vi "VI Tree.vi"() -> ()   [LabVIEW 2017]
uses:
  Private/RegisterVI.vi
  Private/RegisterVIs.vi
  API/JKI Simple Localization.lvlib
panel:
  out "Languages":string[](array[string])
  out "Languages":string[](array[string])
  out "Translated Phrase":string
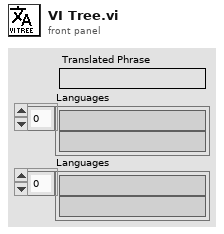
[diagram p1: front panel]
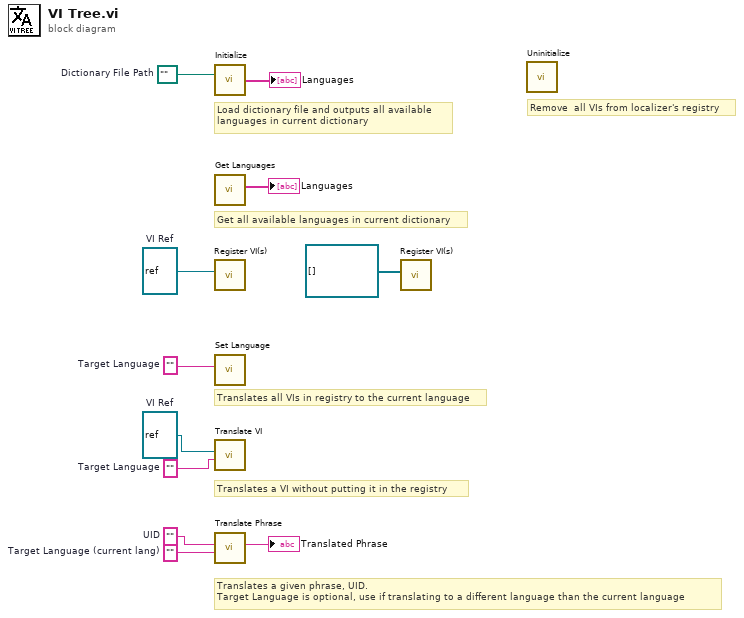
[diagram p0: block diagram]
diagram:
  w1 = ""  # Target Language
  w2 = ""  # Target Language
  w3 = refnum<vi> refnum  # VI Ref
  w4 = path ""  # Dictionary File Path
  w10 = ""  # Target Language (current lang)
  w9 = ""  # UID
  w7 = refnum<vi> refnum  # VI Ref
  # "Translates a VI without putting it in the registry"
  # "Remove  all VIs from localizer's registry"
  # "Translates a given phrase, UID.\nTarget Language is optional, use if translating to a different language than the current language"
  # "Translates all VIs in registry to the current language"
  # "Get all available languages in current dictionary"
  # "Load dictionary file and outputs all available languages in current dictionary"
  n1 = call "Initialize.vi"("Dictionary File Path"=w4) -> ("Languages"=→"Languages":string[])  [unwired: 11 in, 3 out]
  n2 = call "Get Languages.vi"() -> ("Languages"=→"Languages":string[])  [unwired: 10 in, 1 out]
  n3 = call-poly "Register VI(s).vi"("VI Ref"=w7) -> ()  [unwired: 9 in, 2 out]
  n4 = call "Set Language.vi"("Target Language (current lang)"=w1) -> ()  [unwired: 9 in, 2 out]
  n5 = call "Translate VI.vi"("Target Language"=w2, "VI Ref"=w3) -> ()  [unwired: 9 in, 1 out]
  n6 = call "Translate Phrase.vi"("Target Language (current lang)"=w10, "Key"=w9) -> ("Translated Phrase"=→"Translated Phrase":string)  [unwired: 8 in, 1 out]
  n7 = call-poly "Register VI(s).vi"("VI References"=refnum<vi>[] []) -> ()  [unwired: 9 in, 2 out]
  n8 = call "Uninitialize.vi"() -> ()  [unwired: 11 in, 1 out]
